vi "Configurate Channel Osciloscope.vi"(8 "error in (no error)":errorcluster, 10 "Configurate Channel--cluster":T1={"Tektronix"={"Enable Channel (True)"=TRUE, "Channel (0: Channel 1)"=0, "Vertical Coupling (1: DC)"=1, "Probe Attenuation (10: 10X)"=10, "Vertical Range (10.0 V/div)"=10.0, "Vertical Offset (0.0 divs)"=0.0, "Bandwidth (0: MAX Bandwidth)"=0}, "EDU-X-1002A"={"Vertical Scale (5.0 V)"=5.0, "Impedance (0: 1 MOhm)"=0, "Channel Name (0: Channel 1)"=0, "Coupling (1: DC)"=1, "Vertical Range (40.0 V)"=40.0, "Vertical Offset (0.0)"=0.0, "Probe Attenuation (1.0)"=1.0, "Vertical Setting (1: Vertical Range)"=1}} {"EDU-X-1002A"."Vertical Setting (1: Vertical Range)" items=["Vertical Scale", "Vertical Range"]; "EDU-X-1002A"."Coupling (1: DC)" items=["AC", "DC"]; "EDU-X-1002A"."Channel Name (0: Channel 1)" items=["Channel 1", "Channel 2", "Channel 3", "Channel 4"]; "EDU-X-1002A"."Impedance (0: 1 MOhm)" items=["1 MOhm", "50 Ohm"]; "Tektronix"."Bandwidth (0: MAX Bandwidth)" items=["MAX Bandwidth", "Unlimited"]; "Tektronix"."Probe Attenuation (10: 10X)" items=["1"=1, "10"=10, "20"=20, "50"=50, "100"=100, "500"=500, "1000"=1000]; "Tektronix"."Vertical Coupling (1: DC)" items=["AC", "DC", "Ground"]; "Tektronix"."Channel (0: Channel 1)" items=["Channel 1", "Channel 2", "Channel 3", "Channel 4", "Math", "Reference A", "Reference B", "Reference C", "Reference D"]}, 11 "OsciloscopeClass in":refnum<class "OsciloscopeClass.lvclass">) -> (0 "error out":errorcluster, 3 "OsciloscopeClass out":refnum<class "OsciloscopeClass.lvclass">)   [LabVIEW 2020, in "OsciloscopeClass.lvclass"]
uses:
  OsciloscopeClass.lvclass
  TypeDefs/ConfigurateCahnnel--cluster.ctl
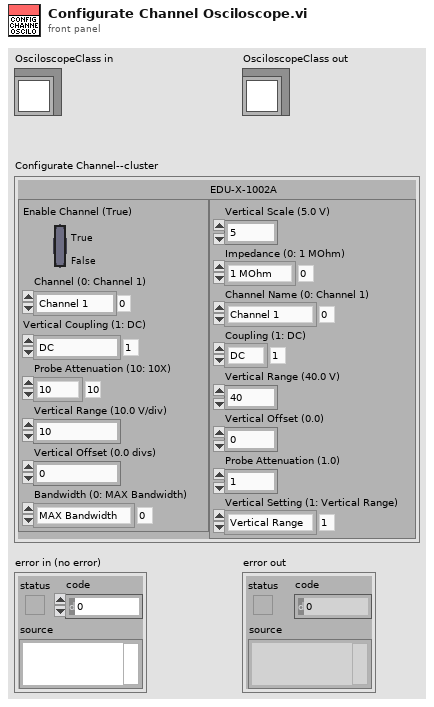
[diagram p1: front panel]
types:
  T1 = typedef "ConfigurateCahnnel--cluster.ctl" = cluster{"Tektronix":cluster{"Enable Channel (True)":bool, "Channel (0: Channel 1)":i32, "Vertical Coupling (1: DC)":i32, "Probe Attenuation (10: 10X)":i32, "Vertical Range (10.0 V/div)":dbl, "Vertical Offset (0.0 divs)":dbl, "Bandwidth (0: MAX Bandwidth)":i32}, "EDU-X-1002A":cluster{"Vertical Scale (5.0 V)":dbl, "Impedance (0: 1 MOhm)":i32, "Channel Name (0: Channel 1)":i32, "Coupling (1: DC)":i32, "Vertical Range (40.0 V)":dbl, "Vertical Offset (0.0)":dbl, "Probe Attenuation (1.0)":dbl, "Vertical Setting (1: Vertical Range)":i32}}
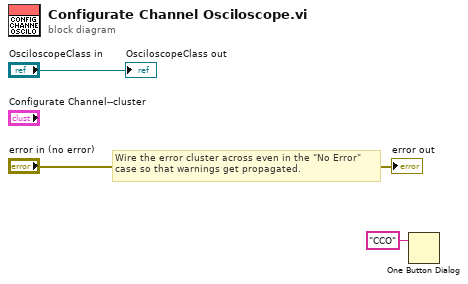
[diagram p0: block diagram]
diagram:
  # "Wire the error cluster across even in the \"No Error\"\ncase so that warnings get propagated."
  n1 = One Button Dialog(message="CCO") -> ()  [unwired: 1 in, 1 out]
  "error out" <- "error in (no error)"
  "OsciloscopeClass out" <- "OsciloscopeClass in"
